vi "LoadGeneralConfigData.vi"(8 "error in (no error)":errorcluster, 11 "configuration file path":path) -> (0 "error out":errorcluster, 3 "Refnum out":T1)   [LabVIEW 2014]
uses:
  <vilib>/Utility/config.llb/Config Data RefNum.ctl
  read/readDoubleKey.vi
  read/readI32.vi
  Variables/Config_Global.vi
  <vilib>/Utility/config.llb/NI_LVConfig.lvlib
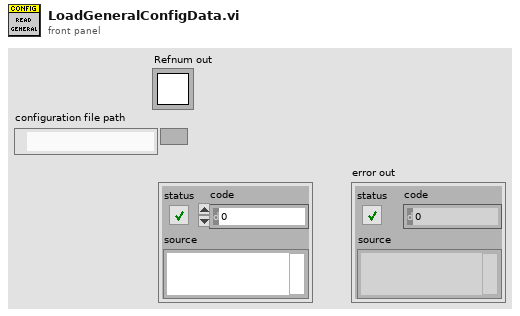
[diagram p1: front panel]
types:
  T1 = typedef "NI_LVConfig.lvlib/Config Data RefNum.ctl" = refnum<k1>
  T2 = cluster{"PodCount":dbl, "PDP_CAN_ID":i32, "PCM_CAN_ID":i32, "BaseRobotMass":dbl, "Warning":string, "error out":errorcluster}
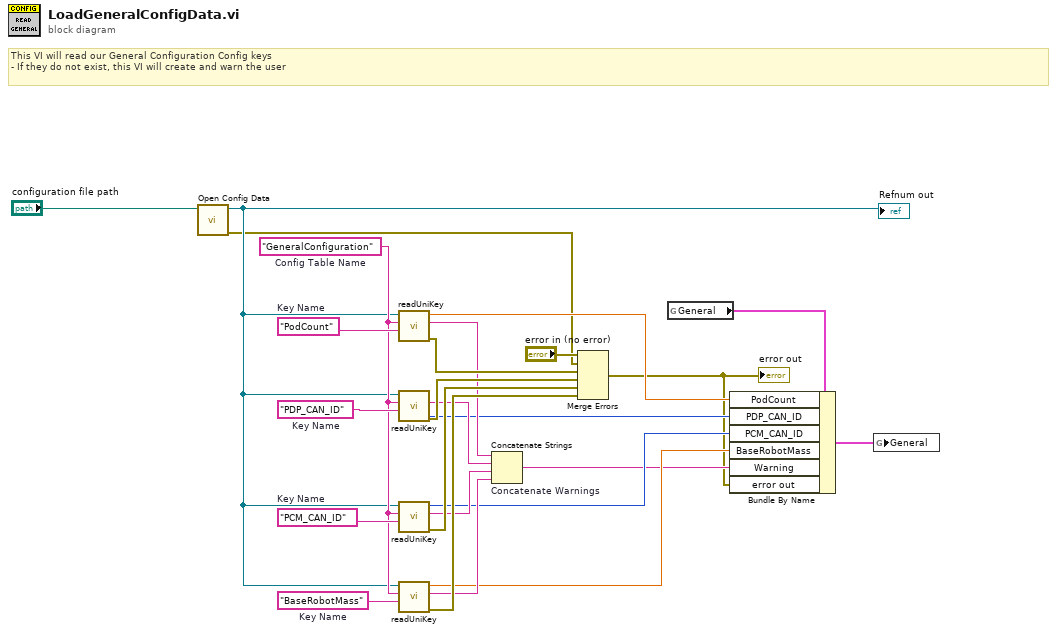
[diagram p0: block diagram]
diagram:
  w22 = "BaseRobotMass"  # Key Name
  w21 = "PCM_CAN_ID"  # Key Name
  w23 = "PDP_CAN_ID"  # Key Name
  w20 = "GeneralConfiguration"  # Config Table Name
  w24 = "PodCount"  # Key Name
  # "This VI will read our General Configuration Config keys\n- If they do not exist, this VI will create and warn the user"
  n1 = call <vilib>:"Open Config Data.vi"("configuration file path"="configuration file path") -> ("error out"=w4:errorcluster, "refnum"=w5:T1)  [unwired: 8 in, 1 out]
  "Refnum out" <- w5
  n2 = call-poly "readUniKey.vi"("Refnum in"=w5, "Section"=w20, "Key Name"=w24) -> ("value"=w10:dbl, "Warning"=w14:string, "error out"=w18:errorcluster)  [unwired: 5 in]
  n3 = call-poly "readUniKey.vi"("Refnum in"=w5, "Section"=w20, "Key Name"=w23) -> ("value"=w9:i32, "Warning"=w13:string, "error out"=w17:errorcluster)  [unwired: 5 in]
  n4 = call-poly "readUniKey.vi"("Refnum in"=w5, "Section"=w20, "Key Name"=w21) -> ("value"=w7:i32, "Warning"=w12:string, "error out"=w16:errorcluster)  [unwired: 5 in]
  n5 = call-poly "readUniKey.vi"("Refnum in"=w5, "Section"=w20, "Key Name"=w22) -> ("value"=w8:dbl, "Warning"=w11:string, "error out"=w15:errorcluster)  [unwired: 5 in]
  n6 = Concatenate Strings "Concatenate Warnings"(w14, w13, w12, w11) -> (w6:string)
  n7 = Merge Errors "Merge Errors"("error in (no error)", w4, w18, w17, w16, w15) -> (w2:errorcluster)
  "error out" <- w2
  n8 = global read "Config_Global.vi" "General"() -> (w3:T2)
  n9 = Bundle By Name(cluster=w3, "PodCount"=w10, "PDP_CAN_ID"=w9, "PCM_CAN_ID"=w7, "BaseRobotMass"=w8, "Warning"=w6, "error out"=w2) -> (w1:T2)
  n10 = global write "Config_Global.vi" "General"(w1) -> ()
